vi "Write Ref.vi"(8 "error in (no error)":errorcluster, 10 "Ref":refnum<visa-resource-name>, 11 "VISA in":refnum<class "VISA.lvclass">) -> (0 "error out":errorcluster, 3 "VISA out":refnum<class "VISA.lvclass">)   [LabVIEW 2023, in "Protocols.lvlib" / "VISA.lvclass"]
uses:
  VISA.lvclass
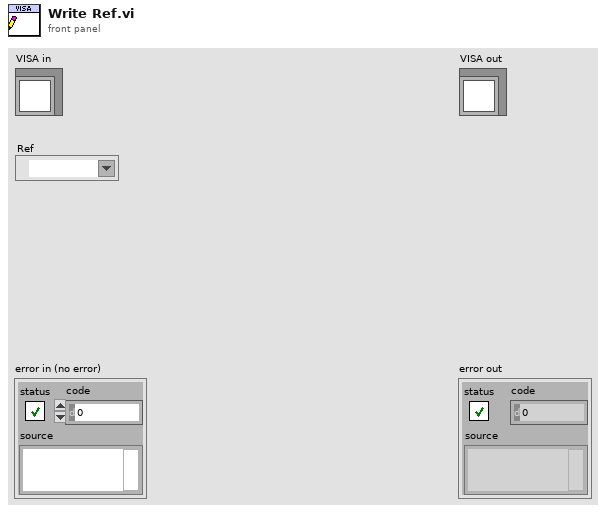
[diagram p1: front panel]
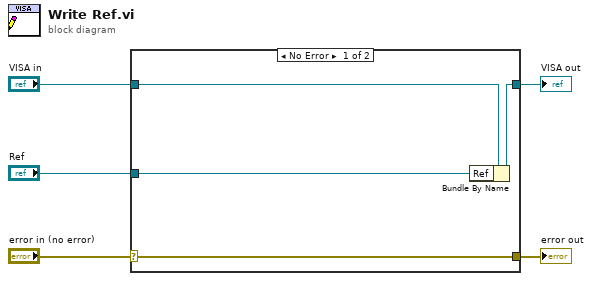
[diagram p0: block diagram]
diagram:
  n1 = case shown="No Error" "error in (no error)" {
    selector: "error in (no error)" -> [w9 w10]
    tunnel: [w9 w10] -> w4
    tunnel: [w7 w11] -> w2
    tunnel: "VISA in" -> [w8 w11]
    tunnel: "Ref" -> [w6 _]
    frame No Error {
      n2 = Bundle By Name(cluster=w8, "Ref"=w6) -> (w7:refnum<class "VISA.lvclass">)
    }
    frame Error {
    }
  }
  "error out" <- w4
  "VISA out" <- w2
